vi "Station Get All.vi"(6 "Descending? (F)":bool, 8 "error in (no error)":errorcluster, 10 "Sort by (sxStationId)":T3, 11 "Connection Refnum":T2) -> (0 "error out":errorcluster, 1 "All Station Instruments":cluster{"Instruments":T1[]}[](array[cluster]), 2 "Station Records":T4[](array[typedef]), 3 "Connection Refnum":T2, 4 "Data Present?":bool)   [LabVIEW 2011]
uses:
  Station Record.ctl
  Station Record Fields.ctl
  Summitek EXT/ODBC/SQL Controls/Connection Refnum.ctl
  Instruments/Instrument Record.ctl
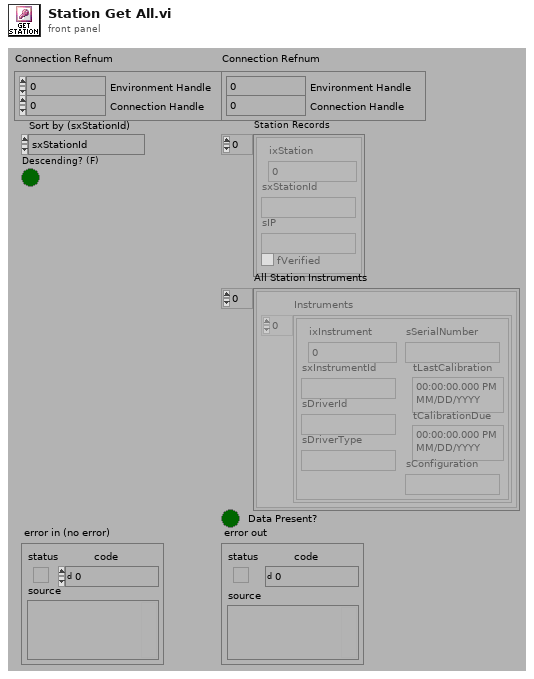
[diagram p1: front panel]
types:
  T1 = typedef "Instrument Record.ctl" = cluster{"ixInstrument":i32, "sxInstrumentId":string, "sDriverId":string, "sDriverType":string, "sSerialNumber":string, "tLastCalibration":timestamp, "tCalibrationDue":timestamp, "sConfiguration":string}
  T2 = typedef "Connection Refnum.ctl" = cluster{"Environment Handle":i32, "Connection Handle":i32}
  T3 = typedef "Station Record Fields.ctl" = enum32{"sxStationId", "sIP", "fVerified", "ixStation"}
  T4 = typedef "Station Record.ctl" = cluster{"ixStation":i32, "sxStationId":string, "sIP":string, "fVerified":bool}
  T5 = typedef "Statement Refnum.ctl" = cluster{"Statement Handle":i32, "Parameter Number":u16}
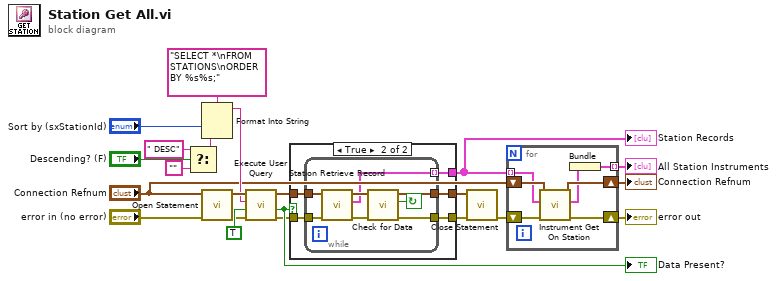
[diagram p0: block diagram]
diagram:
  n1 = Select(t=" DESC" ("input 2"), s="Descending? (F)", f="") -> (s? t:f=w11:string)
  n2 = Format Into String(format string="SELECT *\nFROM STATIONS\nORDER BY %s%s;" ("Query Name"), "Sort by (sxStationId)", w11) -> (resulting string=w14:string)  [unwired: 2 in, 1 out]
  n3 = call "Open Statement.vi"("error in (no error)"="error in (no error)", "Connection Refnum"="Connection Refnum") -> ("error out"=w17:errorcluster, "Statement Refnum"=w18:T5)  [unwired: 4 out]
  n4 = call "Execute User Query.vi"("error in (no error)"=w17, "Return Data? (f)"=TRUE, "User Query"=w14, "Statement Refnum"=w18) -> ("error out"=w21:errorcluster, "Data Present?"=w22:bool, "Statement Refnum"=w20:T5)  [unwired: 1 out]
  "Data Present?" <- w22
  n5 = case shown="True" w22 {
    tunnel: w21 -> [w23 w29]
    tunnel: w20 -> [w24 w28]
    tunnel: [w23 w27] -> w16
    tunnel: [w24 w26] -> w15
    tunnel: [_ w25] -> w3
    frame False {
    }
    frame True {
      n6 = while {
        tunnel: w29 -> [w34]
        tunnel: w28 -> [w31]
        tunnel: [w36] -> w27
        tunnel: [w35] -> w26
        tunnel: [w30] -> w25 mode=indexing
        stop <- w37 continue-if-true
        n7 = call "Station Retrieve Record.vi"("error in (no error)"=w34, "Statement Refnum"=w31) -> ("error out"=w33:errorcluster, "Station Record"=w30:T4, "Statement Refnum"=w32:T5)  [unwired: 7 out]
        n8 = call "Check for Data.vi"("error in (no error)"=w33, "Statement Refnum"=w32) -> ("error out"=w36:errorcluster, "Data Present?"=w37:bool, "Statement Refnum"=w35:T5)  [unwired: 3 out]
      }
    }
  }
  "Station Records" <- w3
  n9 = call "Close Statement.vi"("error in (no error)"=w16, "Statement Refnum"=w15) -> ("error out"=w6:errorcluster)  [unwired: 5 out]
  n10 = for {
    shift-right: [w38] -> w4
    shift-left: w6 -> [w44]
    shift-right: [w42] -> w5
    shift-left: "Connection Refnum" -> [w43]
    tunnel: w3 -> [w41] mode=indexing
    tunnel: [w39] -> w7 mode=indexing
    n11 = call "Instrument Get On Station.vi"("error in (no error)"=w44, "Station Record"=w41, "Connection Refnum"=w43) -> ("error out"=w38:errorcluster, "Instruments on Station"=w40:T1[], "Connection Refnum"=w42:T2)  [unwired: 6 out]
    n12 = Bundle("Instruments on Station"=w40) -> (w39:cluster{"Instruments on Station":T1[]})  [unwired: 1 in]
  }
  "error out" <- w4
  "Connection Refnum" <- w5
  "All Station Instruments" <- w7
